vi "check-sw-env.vi"() -> ()   [LabVIEW 2025]
panel:
  out "UHD response":string
  in  "Python Version":string(combo)="3.10"
  out "Error":errorcluster
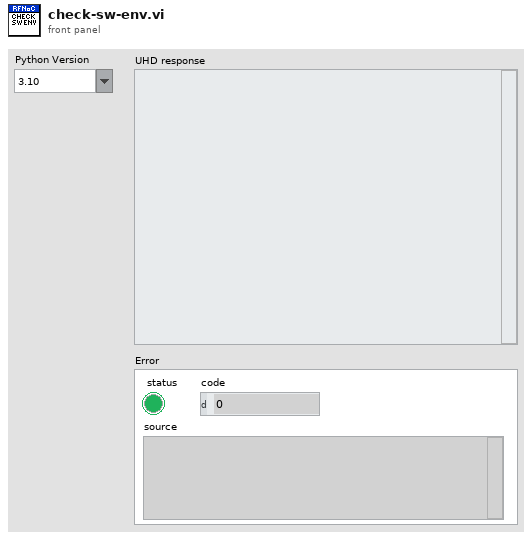
[diagram p1: front panel]
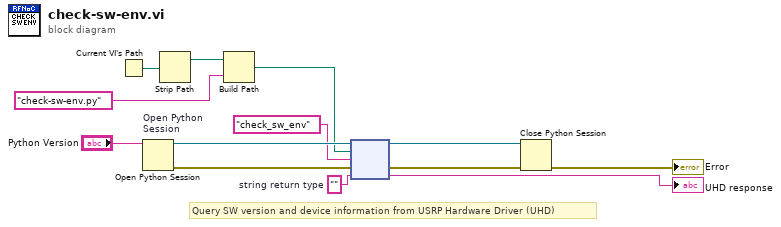
[diagram p0: block diagram]
diagram:
  w2 = ""  # string return type
  # "Query SW version and device information from USRP Hardware Driver (UHD)"
  n1 = Current VI's Path() -> (path=w11:path)
  n2 = Open Python Session "Open Python\nSession"(python version="Python Version") -> (session out=w13:refnum<k35>, error out=w7:errorcluster)  [unwired: 2 in]
  n3 = Strip Path(path=w11) -> (stripped path=w10:path)  [unwired: 1 out]
  n4 = Build Path(base path=w10, name or relative path="check-sw-env.py") -> (appended path=w8:path)
  n5 = node(w13, w8, "check_sw_env" ("function name"), w7, w2) -> (w4:refnum<k35>, w5:errorcluster, →"UHD response":string)  [unwired: 2 out]
  n6 = Close Python Session(session in=w4, error in=w5) -> (11:→"Error":errorcluster)
